vi "Clear Interlock Alarm.vi"(8 "error in":errorcluster, 11 "4124 in":refnum<class "4124.lvclass">) -> (0 "error out":errorcluster, 3 "4124 out":refnum<class "4124.lvclass">)   [LabVIEW 2018, in "4124.lvlib" / "4124.lvclass"]
uses:
  4124.lvclass
  builds/Power_Supply.lvlibp/Power Supply.lvclass
  <instrlib>/NI RMX-412x Power Supplies/NI RMX-412x Power Supplies.lvlib
  C:/Users/Ron.Dexter.LUMINARTECH/Desktop/builds/Power_Supply.lvlibp/Power Supply.lvclass
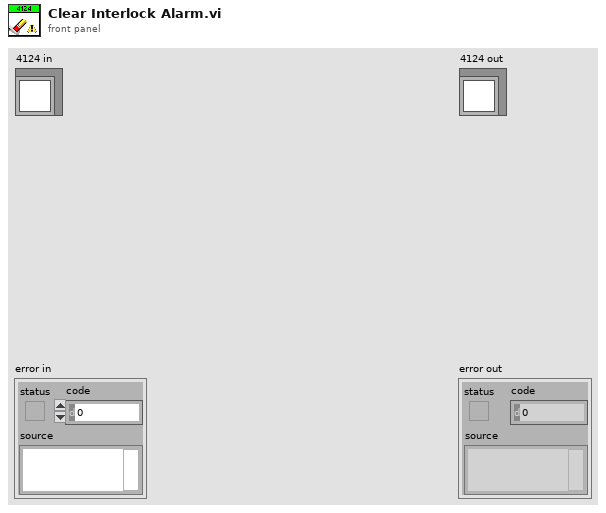
[diagram p1: front panel]
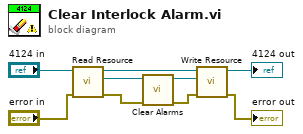
[diagram p0: block diagram]
diagram:
  n1 = call "Read Resource.vi"("error in"="error in", "Power Supply in"="4124 in") -> ("error out"=w2:errorcluster, "Resource"=w4:refnum<visa-resource-name>, "Power Supply out"=w5:refnum<class "4124.lvclass">)  [unwired: 7 in]
  n2 = call <instrlib>:"Clear Alarms.vi"("error in (no error)"=w2, "VISA resource name"=w4) -> ("error out"=w1:errorcluster, "VISA resource name out"=w3:refnum<visa-resource-name>)  [unwired: 8 in]
  n3 = call "Write Resource.vi"("error in"=w1, "Resource"=w3, "Power Supply in"=w5) -> ("error out"=→"error out":errorcluster, "Power Supply out"=→"4124 out":refnum<class "4124.lvclass">)  [unwired: 7 in]
